vi "WPI_GetSetVariantRefNum.vi"(6 "Test Mode Only":bool, 8 "error in (no error)":errorcluster, 9 "Operation":T1, 10 "refnum name":string, 11 "DevRef":variant) -> (0 "error out":errorcluster, 2 "names":string[](array[string]), 3 "DevRef":variant)   [LabVIEW 2017]
doc: "Sets a reference into a registry, gets a reference from a registry, or deletes a reference from a registry. The reference is accessed by name, and can be given any unique name.\n\nThis software is licensed. Open the labview\\readme\\WPI Robotics Library Open Source License.txt file for more information."
uses:
  <vilib>/Rock Robotics/WPI/Utilities/Refnum Registry Operation.ctl
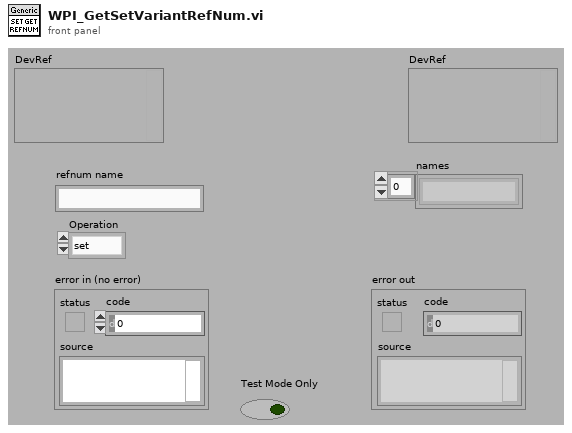
[diagram p1: front panel]
types:
  T1 = typedef "Refnum Registry Operation.ctl" = enum16{"set", "get", "delete", "get all names", "read name"}
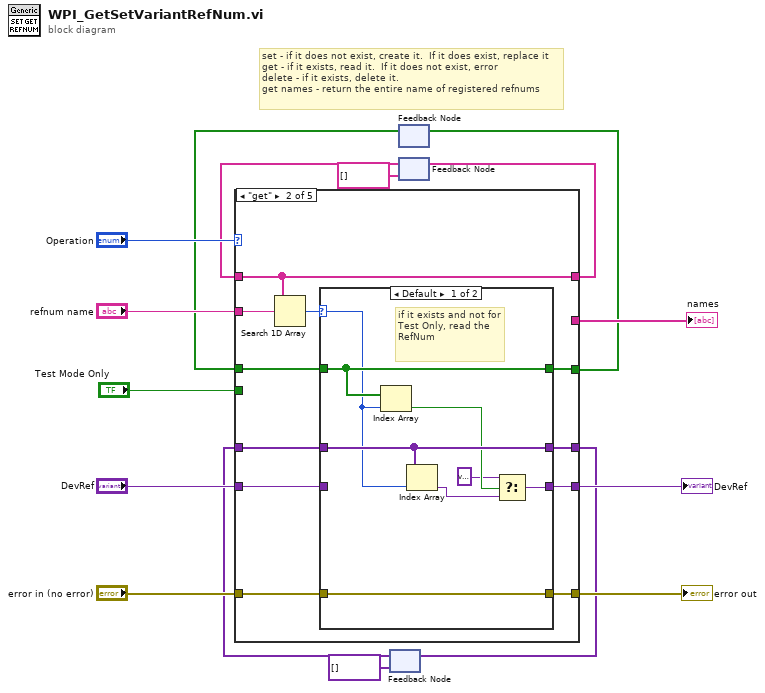
[diagram p0: block diagram]
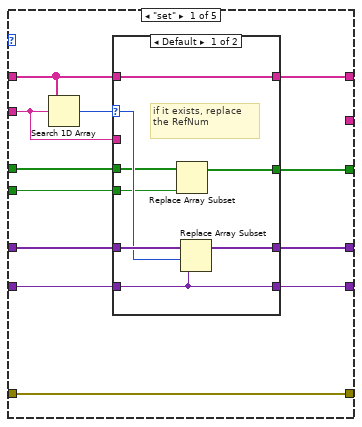
[diagram p2: hidden frame]
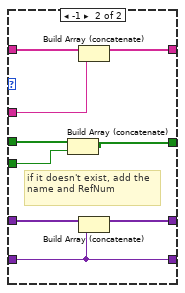
[diagram p3: hidden frame]
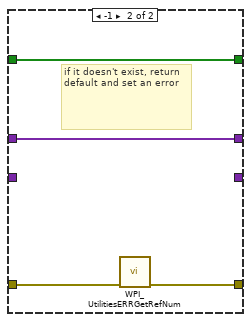
[diagram p4: hidden frame]
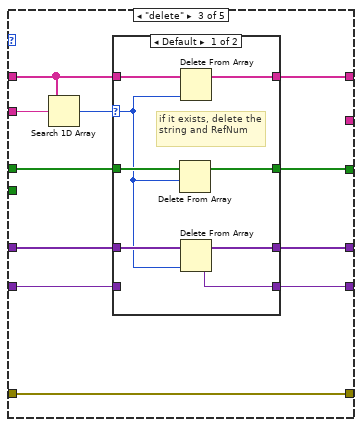
[diagram p5: hidden frame]
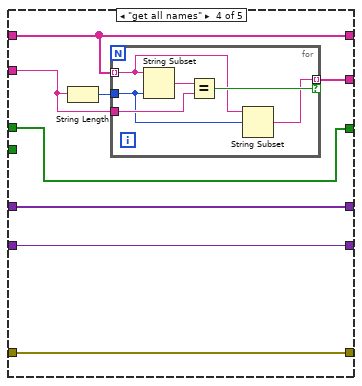
[diagram p7: hidden frame]
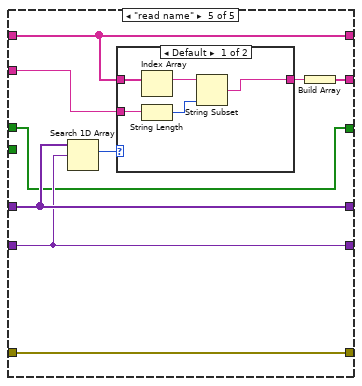
[diagram p8: hidden frame]
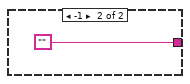
[diagram p9: hidden frame]
diagram:
  # "set - if it does not exist, create it.  If it does exist, replace it\nget - if it exists, read it.  If it does not exist, error\ndelete - if it exists, delete it.\nget names - return the entire name of registered refnums"
  n1 = feedback #1(variant[] []) -> (w8:variant[])
  n2 = feedback #2() -> (w3:bool[])  [unwired: 1 in]
  n3 = feedback #3(string[] []) -> (w6:string[])
  n4 = case shown="\"get\"" "Operation" {
    tunnel: "DevRef" -> [w23 w53 w74 w98 w112]
    tunnel: [w22 w52 w73 w99 w113] -> w9
    tunnel: w8 -> [w24 w54 w75 w99 w113]
    tunnel: [w21 w51 w72 w98 w112] -> w14
    tunnel: [w28 w50 w79 w96 w107] -> w7
    tunnel: w6 -> [w27 w50 w78 w96 w107]
    tunnel: "refnum name" -> [w25 w55 w76 w94 w106]
    tunnel: [w20 w48 w71 w97 w114] -> w12
    tunnel: "error in (no error)" -> [w20 w49 w71 w97 w114]
    tunnel: [_ _ _ w93 w111] -> w10
    tunnel: w3 -> [w19 w47 w70 w92 w110]
    tunnel: [w18 w46 w69 w92 w110] -> w2
    tunnel: "Test Mode Only" -> [w17 _ _ _ _]
    frame "set" {
      n5 = Search 1D Array(1D array=w27, element=w25) -> (index of element=w26:i32)  [unwired: 1 out]
      n6 = case shown="Default" w26 {
        selector: w26 -> [w34 _]
        tunnel: [w36 w45] -> w28
        tunnel: w27 -> [w36 w44]
        tunnel: w25 -> [_ w43]
        tunnel: w24 -> [w35 w42]
        tunnel: w23 -> [w32 w40]
        tunnel: [w33 w41] -> w22
        tunnel: [w32 w40] -> w21
        tunnel: w19 -> [w31 w39]
        tunnel: [w30 w37] -> w18
        tunnel: w17 -> [w29 w38]
        frame Default {
          # "if it exists, replace the RefNum"
          n7 = Replace Array Subset(array=w31, new element=w29) -> (w30:bool[])  [unwired: 1 in]
          n8 = Replace Array Subset(array=w35, new element=w32, index=w34) -> (w33:variant[])
        }
        frame -1 {
          # "if it doesn't exist, add the name and RefNum"
          n9 = Build Array (concatenate)(w39, w38) -> (w37:bool[])
          n10 = Build Array (concatenate)(w44, w43) -> (w45:string[])
          n11 = Build Array (concatenate)(w42, w40) -> (w41:variant[])
        }
      }
    }
    frame "get" {
      n12 = Search 1D Array(1D array=w50, element=w55) -> (index of element=w56:i32)  [unwired: 1 out]
      n13 = case shown="Default" w56 {
        selector: w56 -> [w61 _]
        tunnel: w54 -> [w64 w68]
        tunnel: w53 -> [_ _]
        tunnel: [w64 w68] -> w52
        tunnel: [w60 _] -> w51
        tunnel: w49 -> [w63 w66]
        tunnel: [w63 w67] -> w48
        tunnel: w47 -> [w62 w65]
        tunnel: [w62 w65] -> w46
        frame Default {
          # "if it exists and not for Test Only, read the RefNum"
          n14 = Index Array(array=w62, index=w61) -> (element=w59:bool)
          n15 = Index Array(array=w64, index=w61) -> (element=w57:variant)
          n16 = Select(t=variant ("f"), s=w59, f=w57) -> (s? t:f=w60:variant)
        }
        frame -1 {
          # "if it doesn't exist, return default and set an error"
          n17 = call <vilib>:"WPI_UtilitiesERRGetRefNum.vi"("error in (no error)"=w66) -> ("ERRGetRefNum"=w67:errorcluster)  [unwired: 10 out]
        }
      }
    }
    frame "delete" {
      n18 = Search 1D Array(1D array=w78, element=w76) -> (index of element=w77:i32)  [unwired: 1 out]
      n19 = case shown="Default" w77 {
        selector: w77 -> [w81 _]
        tunnel: [w83 w90] -> w79
        tunnel: w78 -> [w84 w90]
        tunnel: w75 -> [w87 w89]
        tunnel: w74 -> [_ w91]
        tunnel: [w86 w89] -> w73
        tunnel: [w85 w91] -> w72
        tunnel: w70 -> [w82 w88]
        tunnel: [w80 w88] -> w69
        frame Default {
          # "if it exists, delete the string and RefNum"
          n20 = Delete From Array(array=w82, length=w81) -> (array with subset deleted=w80:bool[])  [unwired: 1 in, 1 out]
          n21 = Delete From Array(array=w84, index=w81) -> (array with subset deleted=w83:string[])  [unwired: 1 in, 1 out]
          n22 = Delete From Array(array=w87, index=w81) -> (deleted portion=w85:variant, array with subset deleted=w86:variant[])  [unwired: 1 in]
        }
        frame -1 {
          # "if it doesn't exist, do nothing"
        }
      }
    }
    frame "get all names" {
      n23 = String Length(string=w94) -> (length=w95:i32)
      n24 = for {
        tunnel: w96 -> [w101] mode=indexing
        tunnel: w95 -> [w102]
        tunnel: w94 -> [w103]
        tunnel: [w100] -> w93 mode=indexing if=w104
        n25 = String Subset(string=w101, length (rest)=w102) -> (substring=w105:string)  [unwired: 1 in]
        n26 = Equal?(x=w105, y=w103) -> (x = y?=w104:bool)
        n27 = String Subset(string=w101, offset (0)=w102) -> (substring=w100:string)  [unwired: 1 in]
      }
    }
    frame "read name" {
      n28 = Search 1D Array(1D array=w113, element=w112) -> (index of element=w109:i32)  [unwired: 1 in]
      n29 = case shown="Default" w109 {
        tunnel: [w115 ""] -> w108
        tunnel: w107 -> [w119 _]
        tunnel: w106 -> [w118 _]
        frame Default {
          n30 = Index Array(array=w119) -> (element=w116:string)  [unwired: 1 in]
          n31 = String Length(string=w118) -> (length=w117:i32)
          n32 = String Subset(string=w116, length (rest)=w117) -> (substring=w115:string)  [unwired: 1 in]
        }
        frame -1 {
        }
      }
      n33 = Build Array(w108) -> (w111:string[])
    }
  }
  "error out" <- w12
  "DevRef" <- w14
  "names" <- w10
  n34 = feedback-in #1(w9) -> ()
  n35 = feedback-in #2(w2) -> ()
  n36 = feedback-in #3(w7) -> ()
